vi "Average.vi"(8 "error in (no error)":errorcluster, 10 "Configure":cluster{"start":dbl, "end":dbl, "step":dbl}={"start"=0.05, "end"=0.5, "step"=0.01} {"step" format="%#_6p"; "end" format="%#_6p"; "start" format="%#_6p"}, 11 "Multiple XY-data in":cluster{"X-array":dbl[], "Y-array":dbl[]}[](array[cluster]) {"Y-array" format="%.2p"; "X-array" format="%.2p"}) -> (0 "error out":errorcluster, 3 "Averaged XY-data":cluster{"X-array":dbl[], "Y-array":dbl[]}[](array[cluster]) {"Y-array" format="%.2p"; "X-array" format="%.2p"})   [LabVIEW 2016, in "xy_utilities.lvlib"]
uses:
  <vilib>/Analysis/baseanly.llb/Mean (DBL).vi
  xy_utilities.lvlib
  <vilib>/Analysis/NI_AALBase.lvlib
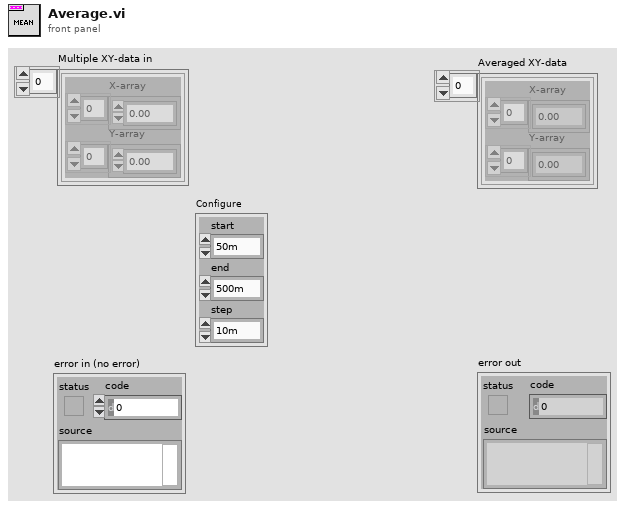
[diagram p1: front panel]
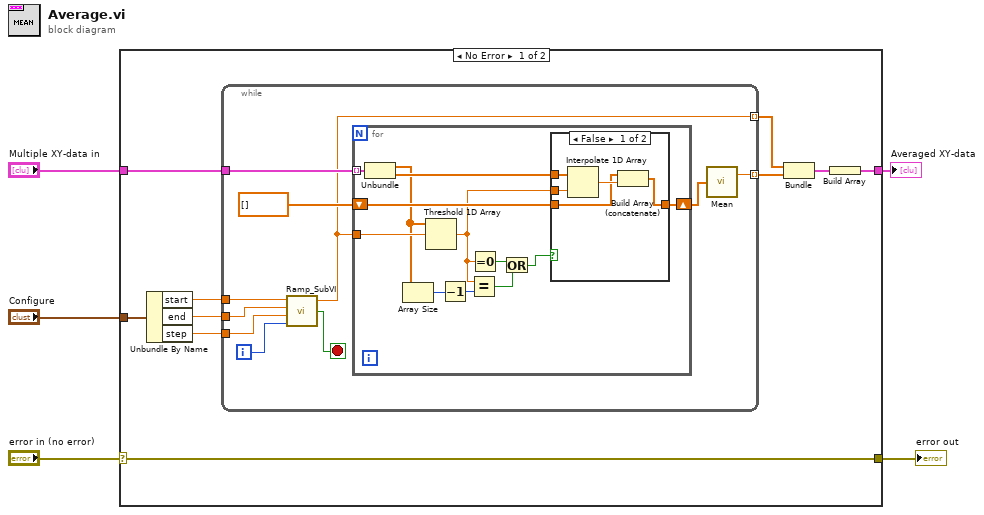
[diagram p0: block diagram]
diagram:
  n1 = case shown="No Error" "error in (no error)" {
    selector: "error in (no error)" -> [w11 w44]
    tunnel: [w13 w45] -> w5
    tunnel: "Multiple XY-data in" -> [w12 w45]
    tunnel: [w11 w44] -> w3
    tunnel: "Configure" -> [w10 _]
    frame No Error {
      n2 = Unbundle By Name(w10) -> ("start"=w9:dbl, "end"=w8:dbl, "step"=w6:dbl)
      n3 = while {
        tunnel: [w24] -> w14 mode=indexing
        tunnel: [w21] -> w7 mode=indexing
        tunnel: w12 -> [w22]
        tunnel: w9 -> [w20]
        tunnel: w8 -> [w19]
        tunnel: w6 -> [w18]
        i -> [w17]
        stop <- w16 stop-if-true
        n4 = call <userlib>:"Ramp_SubVI.vi"("index"=w17, "step"=w18, "end"=w19, "start"=w20) -> ("Stop?"=w16:bool, "Numeric"=w21:dbl)  [unwired: 1 in]
        n5 = for {
          tunnel: w22 -> [w37] mode=indexing
          shift-right: [w36] -> w23
          shift-left: dbl[] [] -> [w35]
          tunnel: w21 -> [w34]
          n6 = Unbundle(w37) -> ("X-array"=w27:dbl[], "Y-array"=w28:dbl[])
          n7 = Array Size(array=w27) -> (size(s)=w30:i32)
          n8 = Threshold 1D Array(2:w34, 3:w27) -> (0:w32:dbl)  [unwired: 1 in]
          n9 = Decrement(x=w30) -> (x-1=w29:i32)
          n10 = Equal?(x=w32, y=w29) -> (x = y?=w31:bool)
          n11 = Equal To 0?(x=w32) -> (x = 0?=w33:bool)
          n12 = Or(x=w33, y=w31) -> (x .or. y?=w26:bool)
          n13 = case shown="False" w26 {
            tunnel: [w40 w43] -> w36
            tunnel: w32 -> [w42 _]
            tunnel: w28 -> [w41 _]
            tunnel: w35 -> [w38 w43]
            frame False {
              n14 = Interpolate 1D Array(1:w42, 2:w41) -> (0:w39:dbl)
              n15 = Build Array (concatenate)(w38, w39) -> (w40:dbl[])
            }
            frame True {
            }
          }
        }
        n16 = call-poly <vilib>:"Mean.vi"("X"=w23) -> ("mean"=w24:dbl)  [unwired: 1 out]
      }
      n17 = Bundle(w7, w14) -> (w15:cluster{dbl[], dbl[]})  [unwired: 1 in]
      n18 = Build Array(w15) -> (w13:cluster{dbl[], dbl[]}[])
    }
    frame Error {
    }
  }
  "Averaged XY-data" <- w5
  "error out" <- w3
